vi "Generate_Interface_Icons.vi"() -> ()   [LabVIEW 2020]
uses:
  <vilib>/picture/picture.llb/imagedata.ctl
panel:
  in  "FolderToSaveImageIn":path=path "c:/Temp/Icons"
  out "new picture 3":picture
  in  "Array 2":string[](array[string])=["Brown", "Burgundy", "Cyan", "DarkBlue", "ForestGreen", "Gray", "Green", "LightGreen", "LightRed", "Pink", "Purple", "Red", "Yellow"]
  in  "Array":u32[](array[colorbox])=[11885056, 6488064, 65504, 3453, 1985280, 11645361, 6618880, 11206513, 16751217, 15335663, 13107311, 14090240, 13025280]
  out "new picture 2":picture
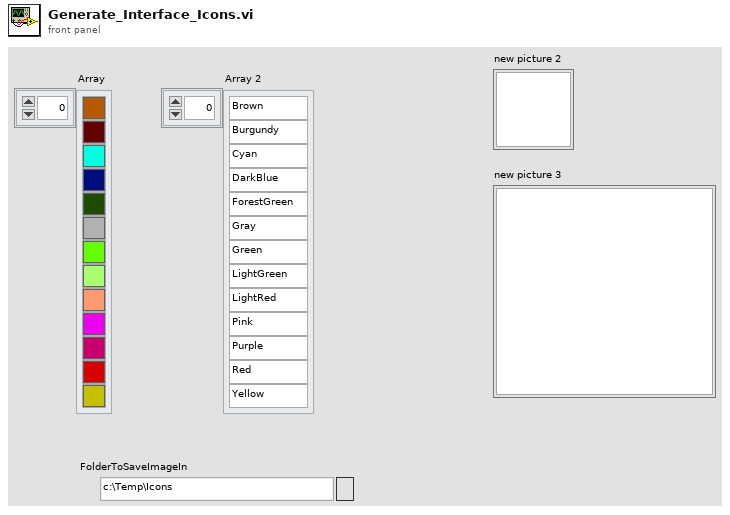
[diagram p1: front panel]
types:
  T1 = typedef "imagedata.ctl" = cluster{"image type":i32, "image depth":i32, "image":u8[], "mask":u8[], "colors":u32[], "Rectangle":cluster{"left":i16, "top":i16, "right":i16, "bottom":i16}}
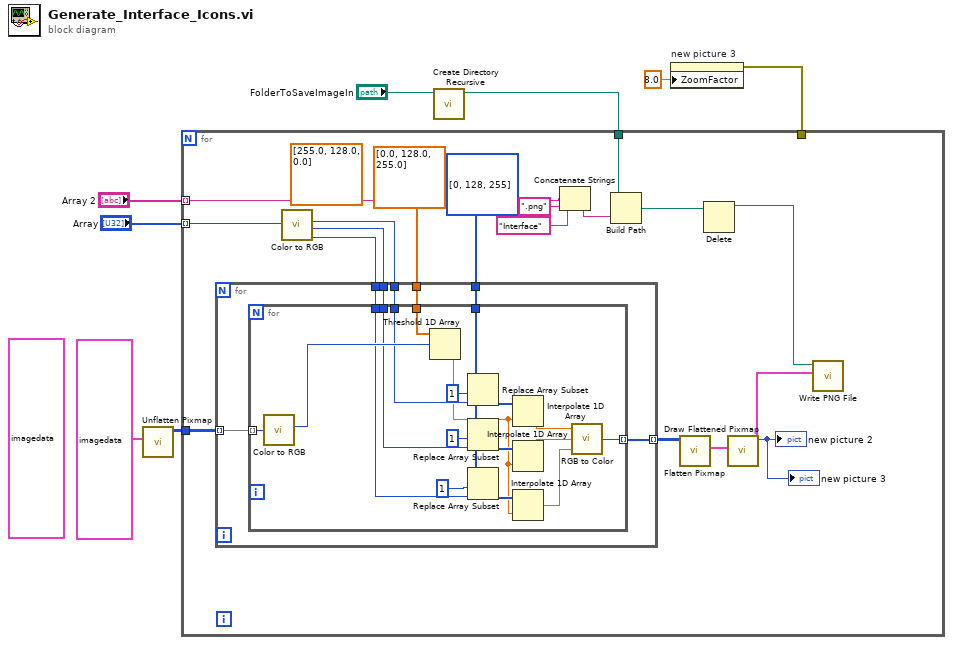
[diagram p0: block diagram]
diagram:
  (unwired) T1 {"image type"=0, "image depth"=24, "image"=[255, 255, 255, 255, 255, 255, 255, 255, 255, 255, 255, 255, 255, 255, 255, 255, 255, 255, 255, 255, 255, 250, 250, 250, 227, 227, 227, 255, 255, 255, 255, 255, 255, 255, 255, 255, 255, 255, 255, 255, 255, 255, 255, 255, 255, 255, 255, 255, 255, 255, 255, 255, 255, 255, 255, 255, 255, 255, 255, 255, 255, 255, 255, 250, 250, 250, 218, 218, 218, 185, 185, 185, 180, 180, 180, 190, 190, 190, 227, 227, 227, 255, 255, 255, 255, 255, 255, 255, 255, 255, 255, 255, 255, 255, 255, 255, 255, 255, 255, 255, 255, 255, 255, 255, 255, 250, 250, 250, 218, 218, 218, 185, 185, 185, 180, 180, 180, 180, 180, 180, 180, 180, 180, 180, 180, 180, 180, 180, 180, 190, 190, 190, 227, 227, 227, 255, 255, 255, 255, 255, 255, 255, 255, 255, 255, 255, 255, 255, 255, 255, 255, 255, 255, 204, 204, 204, 180, 180, 180, 180, 180, 180, 180, 180, 180, 180, 180, 180, 180, 180, 180, 180, 180, 180, 180, 180, 180, 180, 180, 180, 180, 180, 180, 208, 208, 208, 255, 255, 255, 255, 255, 255, 255, 255, 255, 247, 247, 247, 255, 255, 255, 255, 255, 255, 236, 236, 236, 199, 199, 199, 180, 180, 180, 180, 180, 180, 180, 180, 180, 180, 180, 180, 180, 180, 180, 199, 199, 199, 236, 236, 236, 255, 255, 255, 255, 255, 255, 242, 242, 242, 255, 255, 255, 189, 189, 189, 156, 156, 156, 222, 222, 222, 255, 255, 255, 255, 255, 255, 236, 236, 236, 199, 199, 199, 180, 180, 180, 199, 199, 199, 236, 236, 236, 255, 255, 255, 255, 255, 255, 202, 202, 202, 96, 96, 96, 148, 148, 148, 255, 255, 255, 189, 189, 189, 123, 123, 123, 123, 123, 123, 156, 156, 156, 222, 222, 222, 255, 255, 255, 255, 255, 255, 236, 236, 236, 255, 255, 255, 255, 255, 255, 202, 202, 202, 96, 96, 96, 43, 43, 43, 43, 43, 43, 148, 148, 148, 255, 255, 255, 189, 189, 189, 123, 123, 123, 123, 123, 123, 123, 123, 123, 123, 123, 123, 156, 156, 156, 230, 230, 230, 255, 255, 255, 202, 202, 202, 96, 96, 96, 43, 43, 43, 43, 43, 43, 43, 43, 43, 43, 43, 43, 148, 148, 148, 255, 255, 255, 189, 189, 189, 123, 123, 123, 123, 123, 123, 123, 123, 123, 123, 123, 123, 123, 123, 123, 189, 189, 189, 255, 255, 255, 96, 96, 96, 43, 43, 43, 43, 43, 43, 43, 43, 43, 43, 43, 43, 43, 43, 43, 148, 148, 148, 255, 255, 255, 189, 189, 189, 123, 123, 123, 123, 123, 123, 123, 123, 123, 123, 123, 123, 123, 123, 123, 189, 189, 189, 255, 255, 255, 96, 96, 96, 43, 43, 43, 43, 43, 43, 43, 43, 43, 43, 43, 43, 43, 43, 43, 148, 148, 148, 255, 255, 255, 189, 189, 189, 123, 123, 123, 123, 123, 123, 123, 123, 123, 123, 123, 123, 123, 123, 123, 189, 189, 189, 255, 255, 255, 96, 96, 96, 43, 43, 43, 43, 43, 43, 43, 43, 43, 43, 43, 43, 43, 43, 43, 148, 148, 148, 255, 255, 255, 189, 189, 189, 123, 123, 123, 123, 123, 123, 123, 123, 123, 123, 123, 123, 123, 123, 123, 189, 189, 189, 255, 255, 255, 96, 96, 96, 43, 43, 43, 43, 43, 43, 43, 43, 43, 43, 43, 43, 43, 43, 43, 148, 148, 148, 255, 255, 255, 197, 197, 197, 123, 123, 123, 123, 123, 123, 123, 123, 123, 123, 123, 123, 123, 123, 123, 189, 189, 189, 255, 255, 255, 96, 96, 96, 43, 43, 43, 43, 43, 43, 43, 43, 43, 43, 43, 43, 43, 43, 43, 175, 175, 175, 255, 255, 255, 255, 255, 255, 222, 222, 222, 156, 156, 156, 123, 123, 123, 123, 123, 123, 123, 123, 123, 189, 189, 189, 255, 255, 255, 96, 96, 96, 43, 43, 43, 43, 43, 43, 43, 43, 43, 123, 123, 123, 228, 228, 228, 255, 255, 255, 255, 255, 255, 255, 255, 255, 255, 255, 255, 255, 255, 255, 222, 222, 222, 156, 156, 156, 123, 123, 123, 189, 189, 189, 255, 255, 255, 96, 96, 96, 43, 43, 43, 123, 123, 123, 228, 228, 228, 255, 255, 255, 255, 255, 255, 255, 255, 255, 255, 255, 255, 255, 255, 255, 255, 255, 255, 255, 255, 255, 255, 255, 255, 255, 255, 255, 222, 222, 222, 222, 222, 222, 255, 255, 255, 175, 175, 175, 228, 228, 228, 255, 255, 255, 255, 255, 255, 255, 255, 255, 255, 255, 255, 255, 255, 255], "mask"=[255, 255, 255, 255, 255, 255, 255, 255, 255, 255, 255, 255, 255, 255, 255, 255, 255, 255, 255, 255, 255, 255, 255, 255, 255, 255, 255, 255, 255, 255, 255, 255], "colors"=[], "Rectangle"={"left"=0, "top"=0, "right"=16, "bottom"=16}} ("image data")
  n1 = call <vilib>:"Unflatten Pixmap.vi"("image data"=T1 {"image type"=0, "image depth"=24, "image"=array[1152 elements], "mask"=[], "colors"=[], "Rectangle"={"left"=0, "top"=0, "right"=24, "bottom"=16}}) -> ("24-bit pixmap"=w8:u32[][])  [unwired: 4 in, 6 out]
  n2 = call <vilib>:"Create Directory Recursive.vi"("directory"="FolderToSaveImageIn") -> ("directory copy"=w1:path)  [unwired: 4 in, 2 out]
  n3 = property on="new picture 3" class="Pict"("ZoomFactor"=sgl 8.0 ("Zoom Factor")) -> (error out=w4:errorcluster)  [unwired: 2 in, 1 out]
  n4 = for {
    tunnel: w8 -> [w25]
    tunnel: "Array" -> [w23] mode=indexing
    tunnel: "Array 2" -> [w15] mode=indexing
    tunnel: w4 -> [_]
    tunnel: w1 -> [w12]
    (unwired) sgl[] [255.0, 128.0, 0.0]
    n5 = call <vilib>:"Color to RGB.vi"("Color"=w23) -> ("R"=w20:u8, "G"=w21:u8, "B"=w22:u8)  [unwired: 1 out]
    n6 = for {
      tunnel: w25 -> [w32] mode=indexing
      tunnel: [w31] -> w24 mode=indexing
      tunnel: w22 -> [w30]
      tunnel: w21 -> [w29]
      tunnel: w20 -> [w28]
      tunnel: sgl[] [0.0, 128.0, 255.0] -> [w27]
      tunnel: u8[] [0, 128, 255] -> [w26]
      n7 = for {
        tunnel: w32 -> [w50] mode=indexing
        tunnel: [w49] -> w31 mode=indexing
        tunnel: w30 -> [w35]
        tunnel: w29 -> [w36]
        tunnel: w28 -> [w45]
        tunnel: w27 -> [w48]
        tunnel: w26 -> [w38]
        n8 = call <vilib>:"Color to RGB.vi"("Color"=w50) -> ("R"=w47:u8)  [unwired: 3 out]
        n9 = Threshold 1D Array(2:w47, 3:w48) -> (0:w37:sgl)  [unwired: 1 in]
        n10 = Replace Array Subset(array=w38, new element=w45, index=1) -> (w44:u8[])
        n11 = Replace Array Subset(array=w38, new element=w36, index=1) -> (w42:u8[])
        n12 = Replace Array Subset(array=w38, new element=w35, index=1) -> (w39:u8[])
        n13 = Interpolate 1D Array(1:w37, 2:w44) -> (0:w43:dbl)
        n14 = Interpolate 1D Array(1:w37, 2:w42) -> (0:w34:dbl)
        n15 = Interpolate 1D Array(1:w37, 2:w39) -> (0:w33:dbl)
        n16 = call <vilib>:"RGB to Color.vi"("B"=w33, "G"=w34, "R"=w43) -> ("Color"=w49:u32)
      }
    }
    n17 = Concatenate Strings("Interface" ("string"), w15, ".png" ("string")) -> (w13:string)
    n18 = Build Path(base path=w12, name or relative path=w13) -> (appended path=w10:path)
    n19 = call <vilib>:"Flatten Pixmap.vi"("24-bit pixmap"=w24) -> ("image data"=w16:T1)  [unwired: 10 in]
    n20 = Delete(path (use dialog)=w10) -> (deleted path=w9:path)  [unwired: 4 in, 2 out]
    n21 = call <vilib>:"Draw Flattened Pixmap.vi"("image data"=w16) -> ("new picture"=→"new picture 2" →"new picture 3":picture)  [unwired: 8 in]
    n22 = call <vilib>:"Write PNG File.vi"("image data"=w16, "path to PNG file"=w9) -> ()  [unwired: 8 in, 2 out]
  }
